vi "main.vi"() -> ()   [LabVIEW 2014]
uses:
  states.ctl
  key.vi
panel:
  out "Score":u16
  out "NextPos":cluster{"newr":i32, "newc":i32}
  in  "Map":u16[][](array[ring])
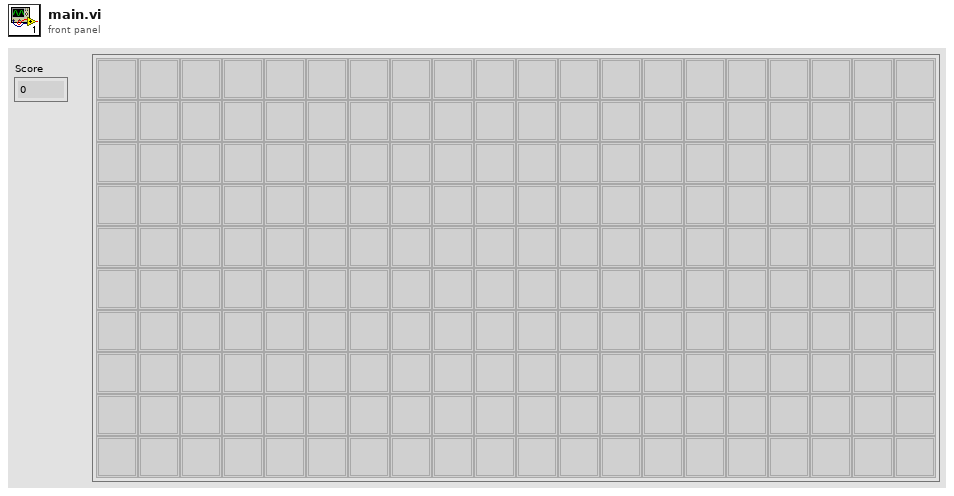
[diagram p1: front panel]
types:
  T1 = typedef "states.ctl" = enum16{"Grow", "GameOver", "Update", "Move", "Collision", "Initialization"}
  T2 = typedef "eventvkey.ctl" = enum16{"ASCII", "Enter", "Return", "Shift", "Ctrl", "Alt", "Cmd", "Opt", "Caps", "NumLock", "Clear", "Break", "Up", "Down", "Left", "Right", "Insert", "Delete", "Home", "End", "PageUp", "PageDown", "Escape", "Help", "Pause", "ScrollLock", "F1", "F2", "F3", "F4", "F5", "F6", "F7", "F8", "F9", "F10", "F11", "F12", "F13", "F14", "F15", "F16", "F17", "F18", "F19", "F20", "F21", "F22", "F23", "F24", "Play", "VolumeUp", "VolumeDown", "Mute", "Two Byte Char"}
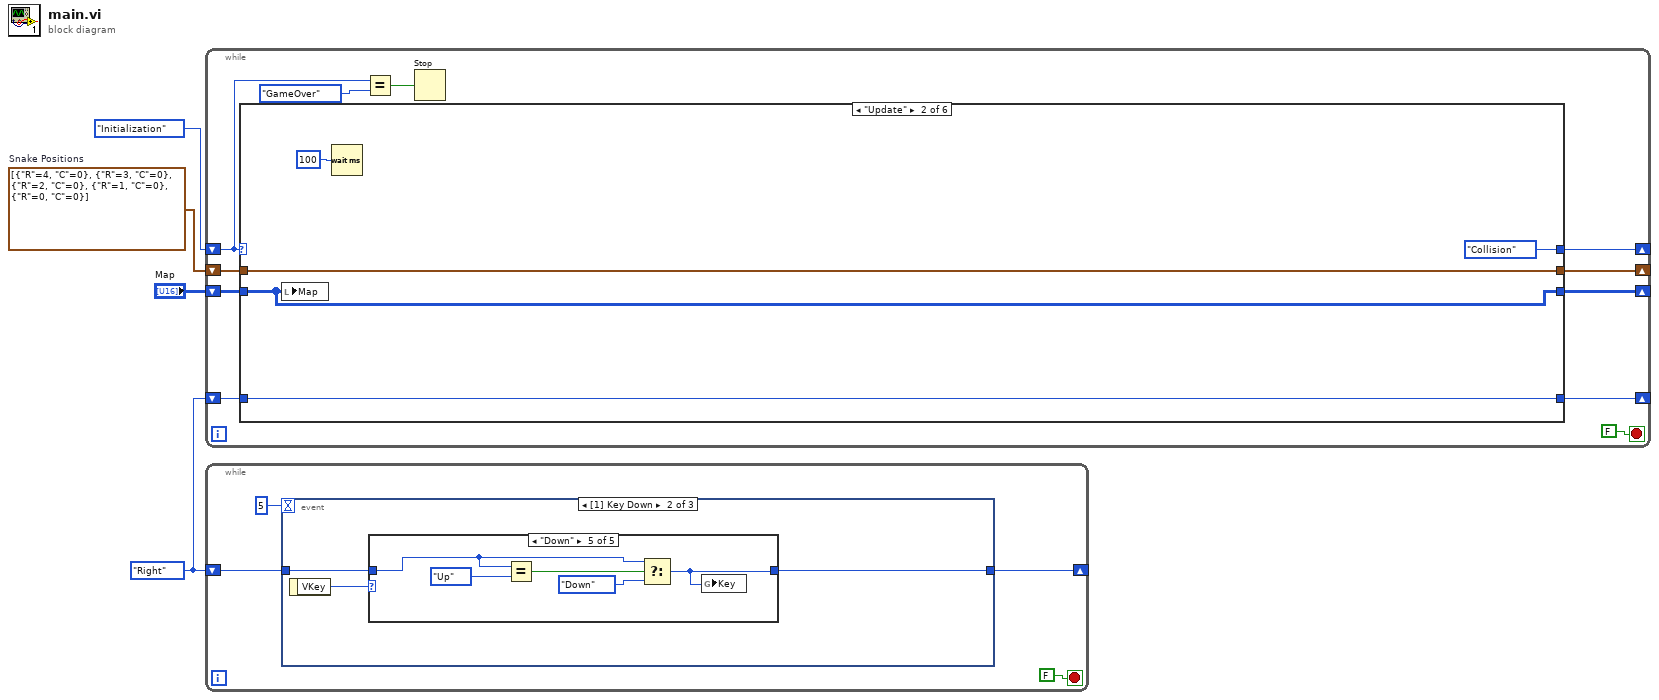
[diagram p0: block diagram]
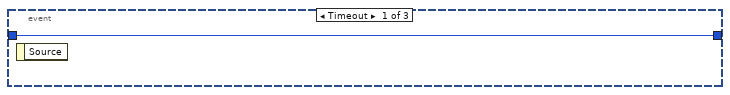
[diagram p2: hidden frame]
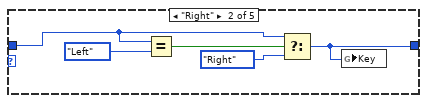
[diagram p4: hidden frame]
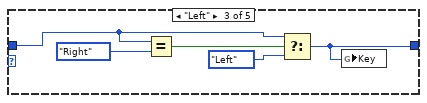
[diagram p5: hidden frame]
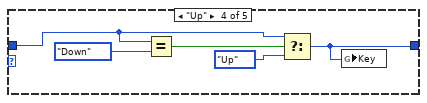
[diagram p6: hidden frame]
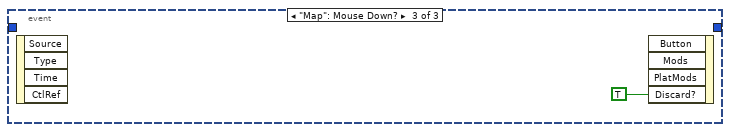
[diagram p7: hidden frame]
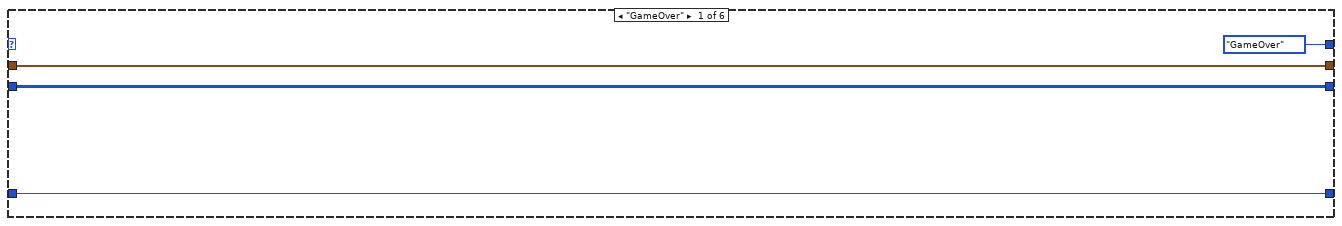
[diagram p8: hidden frame]
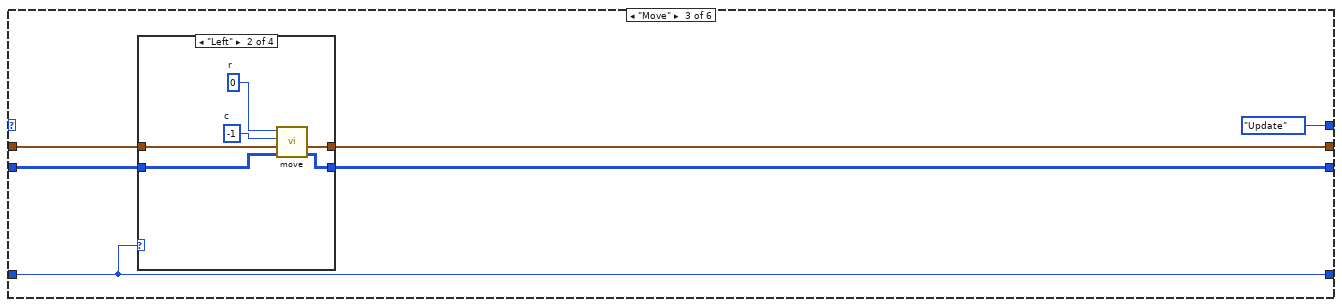
[diagram p9: hidden frame]
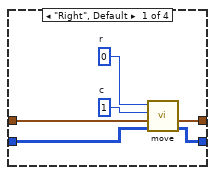
[diagram p10: hidden frame]
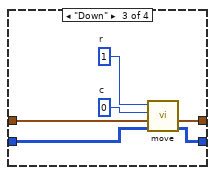
[diagram p11: hidden frame]
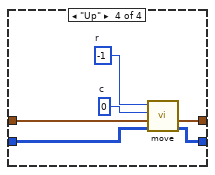
[diagram p12: hidden frame]
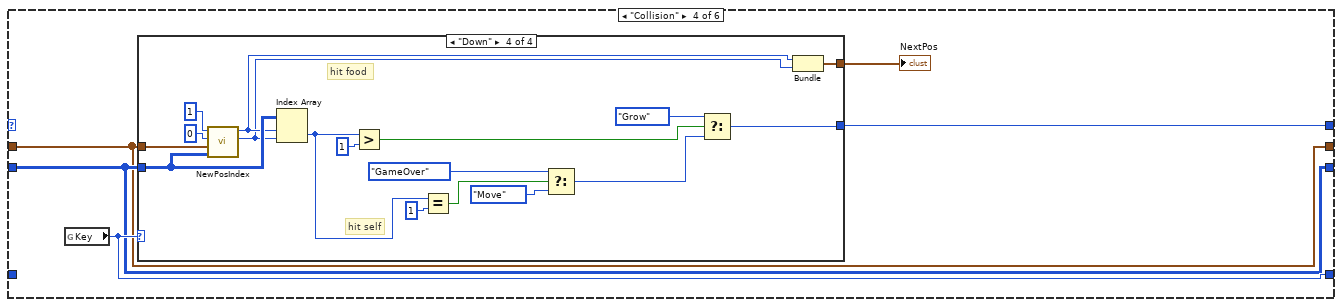
[diagram p13: hidden frame]
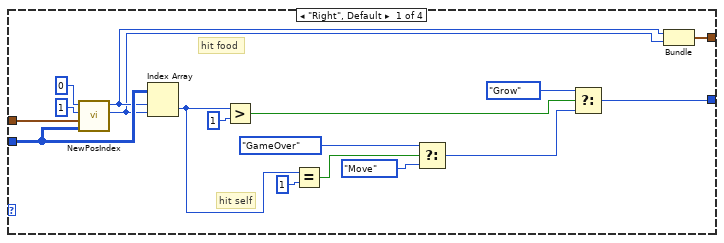
[diagram p14: hidden frame]
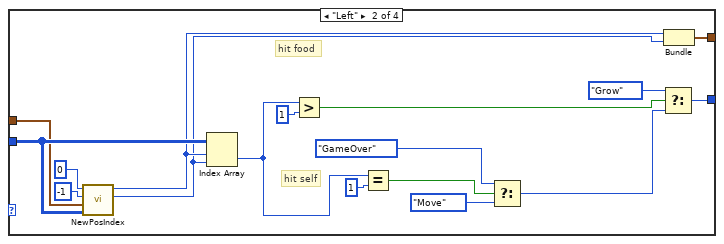
[diagram p15: hidden frame]
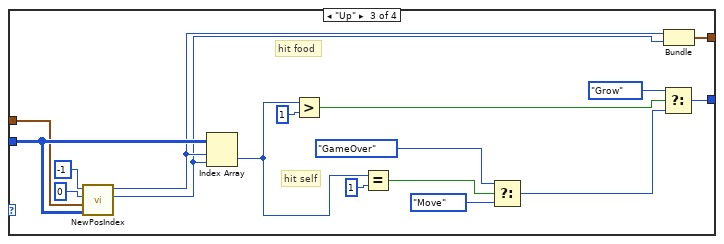
[diagram p16: hidden frame]
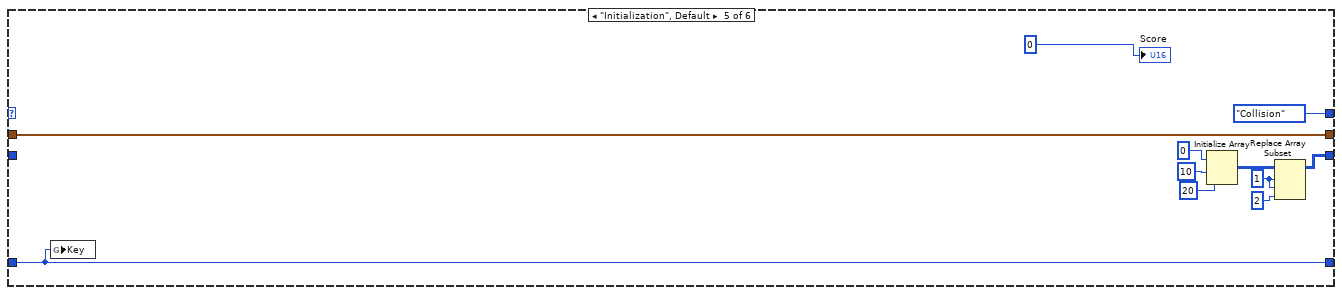
[diagram p17: hidden frame]
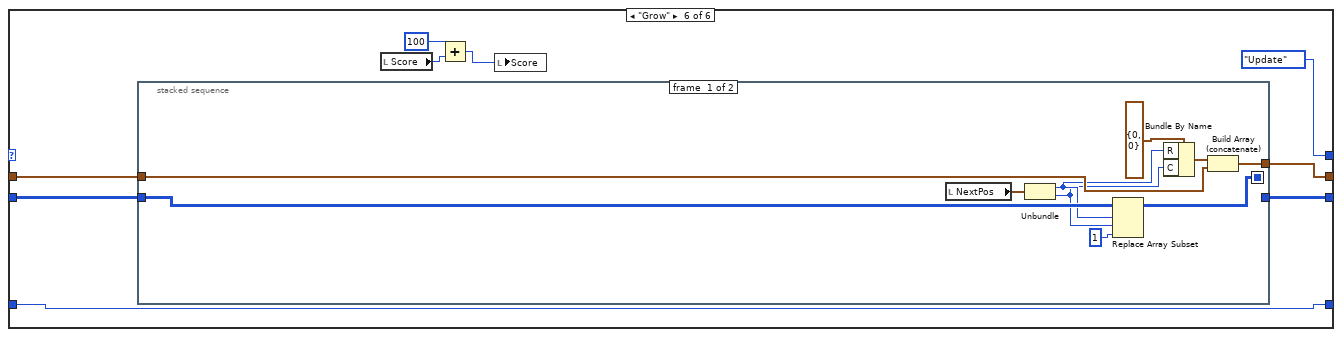
[diagram p18: hidden frame]
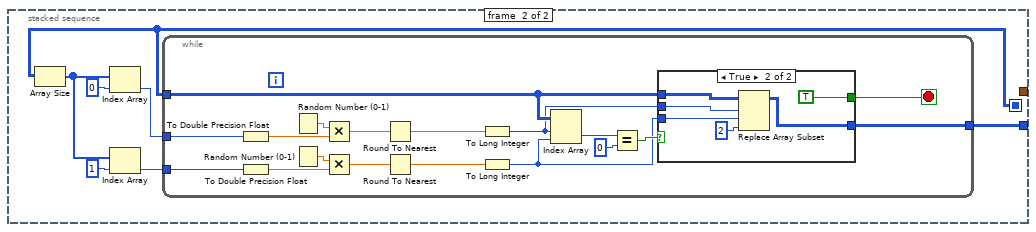
[diagram p19: hidden frame]
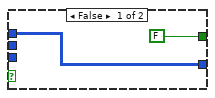
[diagram p20: hidden frame]
diagram:
  w3 = cluster{"R":i32, "C":i32}[] [{"R"=4, "C"=0}, {"R"=3, "C"=0}, {"R"=2, "C"=0}, {"R"=1, "C"=0}, {"R"=0, "C"=0}]  # Snake Positions
  w2 = enum16{"Right", "Left", "Up", "Down"}."Right"
  n1 = while {
    shift-right: [w9] -> _
    shift-left: states."Initialization" -> [w12]
    shift-right: [w5] -> _
    shift-left: "Map" -> [w6]
    shift-right: [w13] -> _
    shift-left: w3 -> [w14]
    shift-right: [w7] -> _
    shift-left: w2 -> [w15]
    stop <- FALSE stop-if-true
    n2 = case shown="\"Update\"" w12 {
      tunnel: w15 -> [w18 w23 w27 _ w136 w146]
      tunnel: w14 -> [w17 w20 w30 w56 w138 w143]
      tunnel: [w17 w20 w29 w56 w138 w142] -> w13
      tunnel: [states."GameOver" states."Collision" states."Update" w58 states."Collision" states."Update"] -> w9
      tunnel: [w18 w23 w27 w59 w136 w146] -> w7
      tunnel: w6 -> [w16 w21 w26 w57 _ w145]
      tunnel: [w16 w21 w25 w57 w130 w144] -> w5
      frame "GameOver" {
      }
      frame "Update" {
        n3 = local write "Map"(w21) -> ()
        n4 = Wait (ms)(milliseconds to wait=u32 100) -> ()  [unwired: 1 out]
      }
      frame "Move" {
        n5 = case shown="\"Left\"" w27 {
          tunnel: w30 -> [w36 w42 w48 w54]
          tunnel: [w33 w39 w45 w51] -> w29
          tunnel: [w32 w38 w44 w50] -> w25
          tunnel: w26 -> [w31 w37 w43 w49]
          frame "Right", Default {
            w34 = 1  # c
            w35 = 0  # r
            n6 = call "move.vi"("Array 4"=w31, "Snake Positions"=w36, "c"=w34, "r"=w35) -> ("Array 5"=w32:u16[][], "Array 2"=w33:cluster{"R":i32, "C":i32}[])  [unwired: 6 in]
          }
          frame "Left" {
            w40 = -1  # c
            w41 = 0  # r
            n7 = call "move.vi"("Array 4"=w37, "Snake Positions"=w42, "c"=w40, "r"=w41) -> ("Array 5"=w38:u16[][], "Array 2"=w39:cluster{"R":i32, "C":i32}[])  [unwired: 6 in]
          }
          frame "Down" {
            w46 = 0  # c
            w47 = 1  # r
            n8 = call "move.vi"("Array 4"=w43, "Snake Positions"=w48, "c"=w46, "r"=w47) -> ("Array 5"=w44:u16[][], "Array 2"=w45:cluster{"R":i32, "C":i32}[])  [unwired: 6 in]
          }
          frame "Up" {
            w52 = 0  # c
            w53 = -1  # r
            n9 = call "move.vi"("Array 4"=w49, "Snake Positions"=w54, "c"=w52, "r"=w53) -> ("Array 5"=w50:u16[][], "Array 2"=w51:cluster{"R":i32, "C":i32}[])  [unwired: 6 in]
          }
        }
      }
      frame "Collision" {
        n10 = global read "key.vi" "Key"() -> (w59:enum16{"Right", "Left", "Up", "Down"})
        n11 = case shown="\"Down\"" w59 {
          tunnel: w57 -> [w64 w81 w98 w115]
          tunnel: [w67 w84 w101 w118] -> w58
          tunnel: w56 -> [w63 w80 w97 w114]
          tunnel: [w60 w77 w96 w111] -> w55
          frame "Right", Default {
            # "hit food"
            # "hit self"
            n12 = call "NewPosIndex.vi"("Array 4"=w64, "Snake Positions"=w63, "c"=1 ("Numeric"), "r"=0 ("Numeric 2")) -> ("newc"=w61:i32, "newr"=w62:i32)  [unwired: 6 in]
            n13 = Index Array(array=w64, index (row)=w62, index (col)=w61) -> (element=w75:u16)
            n14 = Greater?(x=w75, y=u16 1) -> (0:w70:bool)
            n15 = Equal?(x=w75, y=u16 1) -> (x = y?=w73:bool)
            n16 = Select(t=states."GameOver", s=w73, f=states."Move") -> (s? t:f=w68:T1)
            n17 = Select(t=states."Grow", s=w70, f=w68) -> (s? t:f=w67:T1)
            n18 = Bundle("newr"=w62, "newc"=w61) -> (w60:cluster{"newr":i32, "newc":i32})  [unwired: 1 in]
          }
          frame "Left" {
            # "hit food"
            # "hit self"
            n19 = call "NewPosIndex.vi"("Array 4"=w81, "Snake Positions"=w80, "c"=-1 ("Numeric"), "r"=0 ("Numeric 2")) -> ("newc"=w78:i32, "newr"=w79:i32)  [unwired: 6 in]
            n20 = Index Array(array=w81, index (row)=w79, index (col)=w78) -> (element=w92:u16)
            n21 = Greater?(x=w92, y=u16 1) -> (0:w87:bool)
            n22 = Equal?(x=w92, y=u16 1) -> (x = y?=w90:bool)
            n23 = Select(t=states."GameOver", s=w90, f=states."Move") -> (s? t:f=w85:T1)
            n24 = Select(t=states."Grow", s=w87, f=w85) -> (s? t:f=w84:T1)
            n25 = Bundle("newr"=w79, "newc"=w78) -> (w77:cluster{"newr":i32, "newc":i32})  [unwired: 1 in]
          }
          frame "Up" {
            # "hit food"
            # "hit self"
            n26 = call "NewPosIndex.vi"("Array 4"=w98, "Snake Positions"=w97, "c"=0 ("Numeric"), "r"=-1 ("Numeric 2")) -> ("newc"=w94:i32, "newr"=w95:i32)  [unwired: 6 in]
            n27 = Index Array(array=w98, index (row)=w95, index (col)=w94) -> (element=w109:u16)
            n28 = Greater?(x=w109, y=u16 1) -> (0:w104:bool)
            n29 = Equal?(x=w109, y=u16 1) -> (x = y?=w107:bool)
            n30 = Select(t=states."GameOver", s=w107, f=states."Move") -> (s? t:f=w102:T1)
            n31 = Select(t=states."Grow", s=w104, f=w102) -> (s? t:f=w101:T1)
            n32 = Bundle("newr"=w95, "newc"=w94) -> (w96:cluster{"newr":i32, "newc":i32})  [unwired: 1 in]
          }
          frame "Down" {
            # "hit food"
            # "hit self"
            n33 = call "NewPosIndex.vi"("Array 4"=w115, "Snake Positions"=w114, "c"=0 ("Numeric"), "r"=1 ("Numeric 2")) -> ("newc"=w112:i32, "newr"=w113:i32)  [unwired: 6 in]
            n34 = Index Array(array=w115, index (row)=w113, index (col)=w112) -> (element=w126:u16)
            n35 = Greater?(x=w126, y=u16 1) -> (0:w121:bool)
            n36 = Equal?(x=w126, y=u16 1) -> (x = y?=w124:bool)
            n37 = Select(t=states."GameOver", s=w124, f=states."Move") -> (s? t:f=w119:T1)
            n38 = Select(t=states."Grow", s=w121, f=w119) -> (s? t:f=w118:T1)
            n39 = Bundle("newr"=w113, "newc"=w112) -> (w111:cluster{"newr":i32, "newc":i32})  [unwired: 1 in]
          }
        }
        "NextPos" <- w55
      }
      frame "Initialization", Default {
        w132 = 1 ("index (row)")
        n40 = global write "key.vi" "Key"(w136) -> ()
        n41 = Initialize Array(u16 0 ("dimension size"), 10 ("dimension size"), 20 ("dimension size")) -> (w133:u16[][])
        n42 = Replace Array Subset(array=w133, new element=u16 2 ("new element/subarray"), index (row)=w132, index (col)=w132) -> (w130:u16[][])
        "Score" <- u16 0 ("Numeric")
      }
      frame "Grow" {
        n43 = stacked-sequence {
          seq-local: [w154 _] -> [_ w159]
          tunnel: w145 -> [w155 _]
          tunnel: w143 -> [w153 _]
          tunnel: [w148 _] -> w142
          tunnel: [_ w158] -> w144
          frame #0 {
            n44 = local read "NextPos"() -> (w156:cluster{"newr":i32, "newc":i32})
            n45 = Unbundle(w156) -> ("newr"=w151:i32, "newc"=w150:i32)
            n46 = Replace Array Subset(array=w155, new element=u16 1 ("new element/subarray"), index (row)=w151, index (col)=w150) -> (w154:u16[][])
            n47 = Bundle By Name(cluster=cluster{"R":i32, "C":i32} {"R"=0, "C"=0}, "R"=w151, "C"=w150) -> (w149:cluster{"R":i32, "C":i32})
            n48 = Build Array (concatenate)(w149, w153) -> (w148:cluster{"R":i32, "C":i32}[])
          }
          frame #1 {
            n49 = Array Size(array=w159) -> (size(s)=w161:i32[])
            n50 = Index Array(array=w161, index=0) -> (element=w163:i32)
            n51 = Index Array(array=w161, index=1) -> (element=w164:i32)
            n52 = while {
              tunnel: w163 -> [w181]
              tunnel: w164 -> [w179]
              tunnel: w159 -> [w176]
              tunnel: [w172] -> w158
              stop <- w171 stop-if-true
              n53 = To Double Precision Float(number=w181) -> (double precision float=w168:dbl)
              n54 = To Double Precision Float(number=w179) -> (double precision float=w169:dbl)
              n55 = Random Number (0-1)() -> (number: 0 to 1=w167:dbl)
              n56 = Random Number (0-1)() -> (number: 0 to 1=w170:dbl)
              n57 = Multiply(x=w167, y=w168) -> (x*y=w182:dbl)
              n58 = Multiply(x=w170, y=w169) -> (x*y=w180:dbl)
              n59 = Round To Nearest(number=w182) -> (nearest integer value=w175:dbl)
              n60 = Round To Nearest(number=w180) -> (nearest integer value=w174:dbl)
              n61 = To Long Integer(number=w175) -> (32bit integer=w166:i32)
              n62 = To Long Integer(number=w174) -> (32bit integer=w165:i32)
              n63 = Index Array(array=w176, index (row)=w166, index (col)=w165) -> (element=w178:u16)
              n64 = Equal?(x=w178, y=u16 0 ("x")) -> (x = y?=w173:bool)
              n65 = case shown="True" w173 {
                tunnel: w176 -> [w184 w190]
                tunnel: w166 -> [_ w189]
                tunnel: w165 -> [_ w188]
                tunnel: [w184 w186] -> w172
                tunnel: [FALSE TRUE] -> w171
                frame False {
                }
                frame True {
                  n66 = Replace Array Subset(array=w190, new element=u16 2 ("new element/subarray"), index (row)=w189, index (col)=w188) -> (w186:u16[][])
                }
              }
            }
          }
        }
        n67 = local read "Score"() -> (w140:u16)
        n68 = Add(x=u16 100, y=w140) -> (x+y=w141:u16)
        n69 = local write "Score"(w141) -> ()
      }
    }
    n70 = Equal?(x=w12, y=states."GameOver") -> (x = y?=w10:bool)
    n71 = Stop(stop? (T)=w10) -> ()
  }
  n72 = while {
    shift-right: [w192] -> _
    shift-left: w2 -> [w193]
    stop <- FALSE stop-if-true
    n73 = event shown="[1] Key Down" {
      selector: _ -> [_ _ _]
      dyn-events: _ -> [_ _ _]
      timeout: 5 -> [_ _ _]
      tunnel: w193 -> [w195 w196 _]
      tunnel: [w195 w197 _] -> w192
      event Timeout {
        n74 = event-data() -> ()  [unwired: 1 in, 1 out]
      }
      event Key Down {
        n75 = event-data() -> ("VKey"=w198:T2)  [unwired: 1 in]
        n76 = case shown="\"Down\"" w198 {
          tunnel: [w199 w201 w206 w211 w216] -> w197
          tunnel: w196 -> [w199 w203 w208 w213 w218]
          frame "Insert", Default {
          }
          frame "Right" {
            n77 = Equal?(x=w203, y=enum16{"Right", "Left", "Up", "Down"}."Left") -> (x = y?=w204:bool)
            n78 = Select(t=w203, s=w204, f=enum16{"Right", "Left", "Up", "Down"}."Right") -> (s? t:f=w201:enum16{"Right", "Left", "Up", "Down"})
            n79 = global write "key.vi" "Key"(w201) -> ()
          }
          frame "Left" {
            n80 = Equal?(x=w208, y=enum16{"Right", "Left", "Up", "Down"}."Right") -> (x = y?=w209:bool)
            n81 = Select(t=w208, s=w209, f=enum16{"Right", "Left", "Up", "Down"}."Left") -> (s? t:f=w206:enum16{"Right", "Left", "Up", "Down"})
            n82 = global write "key.vi" "Key"(w206) -> ()
          }
          frame "Up" {
            n83 = Equal?(x=w213, y=enum16{"Right", "Left", "Up", "Down"}."Down") -> (x = y?=w214:bool)
            n84 = Select(t=w213, s=w214, f=enum16{"Right", "Left", "Up", "Down"}."Up") -> (s? t:f=w211:enum16{"Right", "Left", "Up", "Down"})
            n85 = global write "key.vi" "Key"(w211) -> ()
          }
          frame "Down" {
            n86 = Equal?(x=w218, y=enum16{"Right", "Left", "Up", "Down"}."Up") -> (x = y?=w219:bool)
            n87 = Select(t=w218, s=w219, f=enum16{"Right", "Left", "Up", "Down"}."Down") -> (s? t:f=w216:enum16{"Right", "Left", "Up", "Down"})
            n88 = global write "key.vi" "Key"(w216) -> ()
          }
        }
      }
      event "Map": Mouse Down? {
        n89 = event-data() -> ()  [unwired: 1 in, 4 out]
        n90 = event-data("Discard?"=TRUE) -> ()  [unwired: 4 in, 1 out]
      }
    }
  }
